vi "Compute Peak SPL.vi"(0 "Waveform Class":refnum<class "Waveform Class.lvclass">=refnum, 5 "Speaker or side":string, 11 "error in (no error)":errorcluster) -> (4 "Peak SPL":dbl, 15 "error out":errorcluster)   [LabVIEW 2015]
uses:
  Signal Generation VIs/Waveform Classes/Waveform Class.lvclass
  <vilib>/Analysis/NI_AALPro.lvlib
  <vilib>/Analysis/2dsp.llb/Inverse Complex FFT.vi
  Utility VIs/Math VIs/Linear to dB (scalar).vi
panel:
  out "Waveform Graph":dbl[](graph)
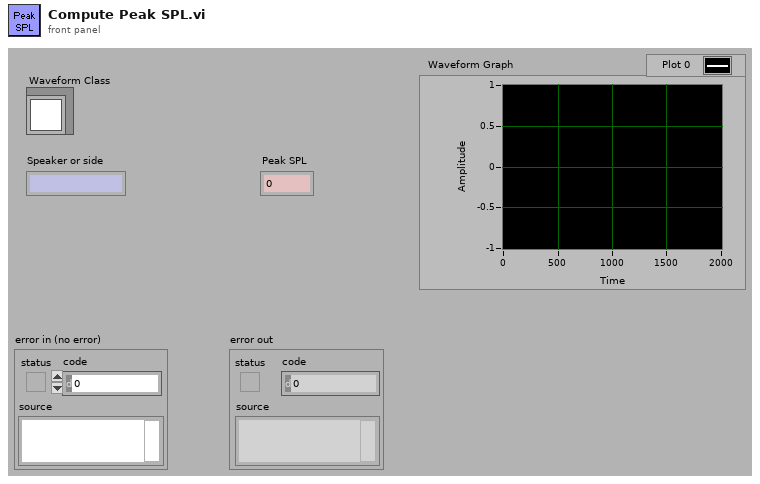
[diagram p1: front panel]
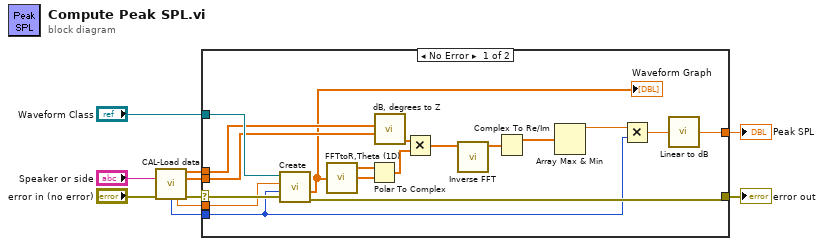
[diagram p0: block diagram]
diagram:
  n1 = call "CAL-Load data.vi"(5:"Speaker or side", "error in (no error)"="error in (no error)") -> ("Frequency (Hz)"=w7:dbl[], "Mag"=w5:dbl[], "npts"=w2:i32, "Fs (Hz)"=w3:dbl, "error out"=w9:errorcluster)  [unwired: 6 in, 3 out]
  n2 = case shown="No Error" w9 {
    selector: w9 -> [w27 w29]
    tunnel: [w25 w29] -> w8
    tunnel: w7 -> [w17 _]
    tunnel: w5 -> [w16 _]
    tunnel: "Waveform Class" -> [w28 _]
    tunnel: w3 -> [w26 _]
    tunnel: w2 -> [w14 _]
    tunnel: [w21 _] -> w1
    frame No Error {
      n3 = call-dynamic "Create.vi"("error in (no error)"=w27, "Npts"=w14, "Sampling Rate (Hz)"=w26, "Waveform Class in"=w28) -> ("error out"=w25:errorcluster, "Waveform"=w11:dbl[])  [unwired: 4 in, 2 out]
      "Waveform Graph" <- w11
      n4 = call "FFTtoR,Theta (1D).VI"("X"=w11) -> ("+Freq. Mag of FFT"=w18:dbl[], "+Freq Theta of FFT"=w24:dbl[])  [unwired: 1 in]
      n5 = Polar To Complex(1:w24, 2:w18) -> (0:w23:cdb[])
      n6 = call "dB, degrees to Z.vi"("Phase (degrees)"=w16, "Magnitude (dB)"=w17) -> ("Z"=w20:cdb[])  [unwired: 2 in]
      n7 = Multiply(x=w20, y=w23) -> (x*y=w19:cdb[])
      n8 = call-poly <vilib>:"Inverse FFT.vi"("FFT {X}"=w19) -> ("X"=w22:cdb[])  [unwired: 9 in, 1 out]
      n9 = Complex To Re/Im(x + iy=w22) -> (x=w15:dbl[])  [unwired: 1 out]
      n10 = Array Max & Min(array=w15) -> (max value=w12:dbl)  [unwired: 3 out]
      n11 = Multiply(x=w12, y=w14) -> (x*y=w13:dbl)
      n12 = call-poly "Linear to dB.vi"("Linear"=w13) -> ("dB"=w21:dbl)
    }
    frame Error {
    }
  }
  "error out" <- w8
  "Peak SPL" <- w1
